vi "PDHydra - PWM_v2.vi"(8 "error in":errorcluster, 9 "Board Selector":T1, 10 "HMP VISA":refnum<visa-resource-name>="HMP4040_FTS2", 11 "ControlBoardVISA":refnum<visa-resource-name>="ControlBoard") -> (0 "error out":errorcluster, 1 "50% Duty Cycle":dbl[](array[numeric]), 2 "25% Duty":dbl[](array[numeric]), 3 "0% Duty":dbl[](array[numeric]))   [LabVIEW 2022 SP3]
uses:
  Serial Board Com/Board Select.ctl
  Serial Board Com/ADCSelector BB.ctl
  HMP4000 Communication/HMP4040_ChannelControlAutomatic.ctl
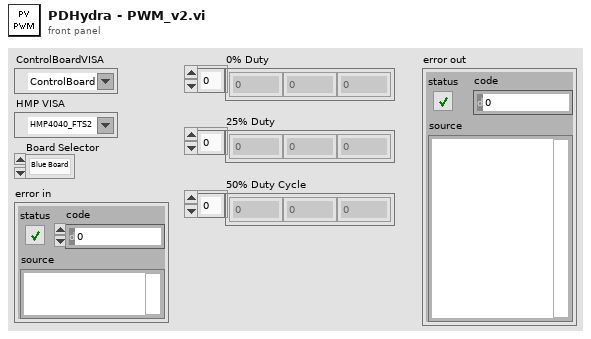
[diagram p1: front panel]
types:
  T1 = typedef "Board Select.ctl" = enum16{"Blue Board", "Green Board"}
  T2 = typedef "HMP4040_ChannelControlAutomatic.ctl" = enum16{"Off", "Control Power", "HMP2020 Control + DC32V", "HMP2020 Control + DC8V", "HMP4040 Control + DC32V", "HMP4040 Control +DC8V", "HMP4040 Ch2 24V 4A"}
  T3 = typedef "ADCSelector BB.ctl" = enum16{"INVA_ISENSE_U", "INVA_ISENSE_V", "INVA_ISENSE_W", "INVA_UDC", "INVA_TEMP", "HB_TEMP", "AUXB_TEMP", "VLINE_AB", "VLINE_BC", "VLINE_CA", "VSENSE_POS_24V", "VSENSE_POS_5V", "VSENSE_NEG_15V", "INVB_ISENSE_U", "INV_B_ISENSEV", "INVB_ISENSE_W", "INVB_UDC", "INVB_TEMP", "AUXA_TEMP", "AUXC_TEMP", "VOUT_AB", "VOUT_BC", "VOUT_CA", "VSENSE_POS_15V", "VSENSE_POS_3P3V", "TEST_POINT"}
  T4 = cluster{"Enum":T3, "Duty Cycle On":i32, "Leg":i32, "Duty Cycle Off":i32}[]
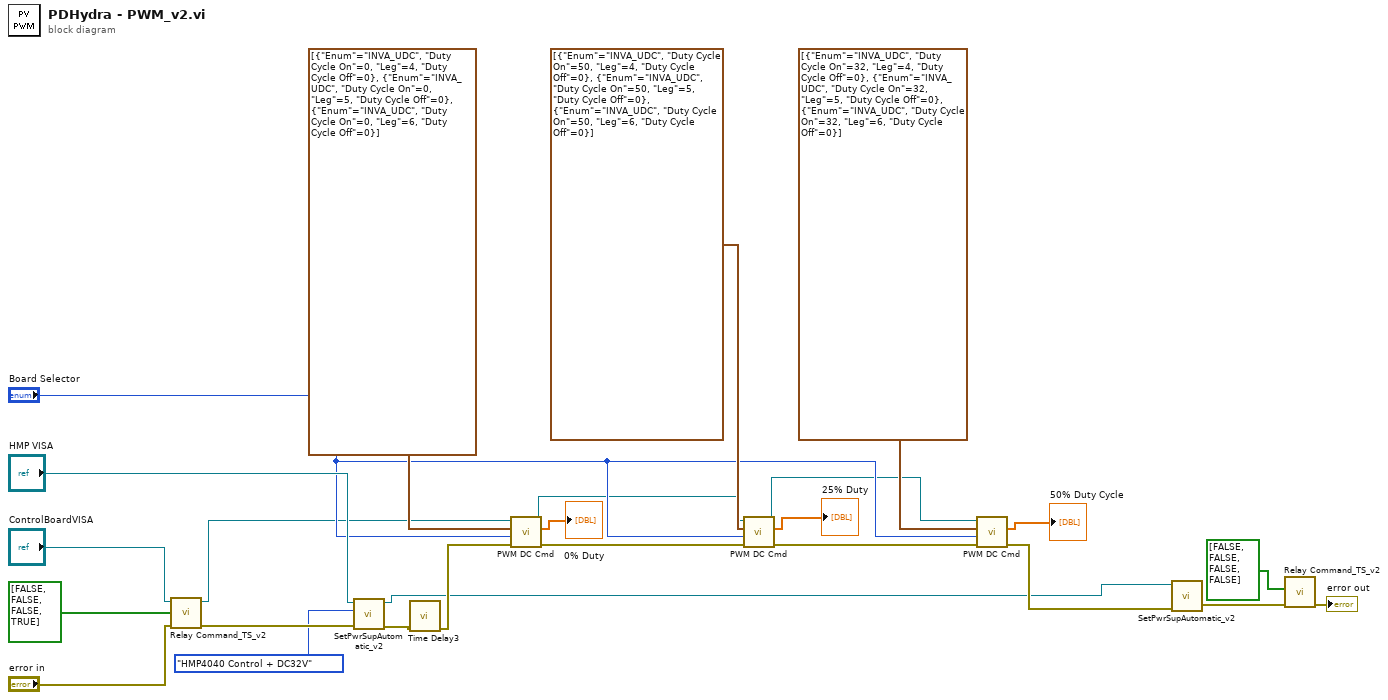
[diagram p0: block diagram]
diagram:
  n1 = call "Relay Command_TS_v2.vi"("error in (no error)"="error in", "Relay Command"=bool[] [FALSE, FALSE, FALSE, TRUE], "Control Board VISA"="ControlBoardVISA") -> ("error out"=w22:errorcluster, "VISA Refnum out"=w8:refnum<visa-resource-name>)  [unwired: 7 in]
  n2 = call "SetPwrSupAutomatic_v2.vi"("error in (no error)"=w22, "Enum"=HMP4040_ChannelControlAutomatic."HMP4040 Control + DC32V", "HMP VISA"="HMP VISA") -> ("error out"=w21:errorcluster, "HMP VISA Out"=w7:refnum<visa-resource-name>)  [unwired: 7 in]
  n3 = call "Time Delay3"("error in (no error)"=w21) -> ("error out"=w17:errorcluster)  [unwired: 10 in]
  n4 = call "PWM DC Cmd.vi"("error in (no error)"=w17, "Board Selector"="Board Selector", "Array in"=T4 [{"Enum"=enum."INVA_UDC", "Duty Cycle On"=0, "Leg"=4, "Duty Cycle Off"=0}, {"Enum"=enum."INVA_UDC", "Duty Cycle On"=0, "Leg"=5, "Duty Cycle Off"=0}, {"Enum"=enum."INVA_UDC", "Duty Cycle On"=0, "Leg"=6, "Duty Cycle Off"=0}], "VISA Refnum in"=w8) -> ("error out"=w19:errorcluster, "Array out"=→"0% Duty":dbl[], "VISA Refnum out"=w4:refnum<visa-resource-name>)  [unwired: 5 in]
  n5 = call "PWM DC Cmd.vi"("error in (no error)"=w19, "Board Selector"="Board Selector", "Array in"=T4 [{"Enum"=enum."INVA_UDC", "Duty Cycle On"=50, "Leg"=4, "Duty Cycle Off"=0}, {"Enum"=enum."INVA_UDC", "Duty Cycle On"=50, "Leg"=5, "Duty Cycle Off"=0}, {"Enum"=enum."INVA_UDC", "Duty Cycle On"=50, "Leg"=6, "Duty Cycle Off"=0}], "VISA Refnum in"=w4) -> ("error out"=w15:errorcluster, "Array out"=→"25% Duty":dbl[], "VISA Refnum out"=w3:refnum<visa-resource-name>)  [unwired: 5 in]
  n6 = call "PWM DC Cmd.vi"("error in (no error)"=w15, "Board Selector"="Board Selector", "Array in"=T4 [{"Enum"=enum."INVA_UDC", "Duty Cycle On"=32, "Leg"=4, "Duty Cycle Off"=0}, {"Enum"=enum."INVA_UDC", "Duty Cycle On"=32, "Leg"=5, "Duty Cycle Off"=0}, {"Enum"=enum."INVA_UDC", "Duty Cycle On"=32, "Leg"=6, "Duty Cycle Off"=0}], "VISA Refnum in"=w3) -> ("error out"=w11:errorcluster, "Array out"=→"50% Duty Cycle":dbl[])  [unwired: 5 in, 1 out]
  n7 = call "SetPwrSupAutomatic_v2.vi"("error in (no error)"=w11, "HMP VISA"=w7) -> ("error out"=w14:errorcluster)  [unwired: 8 in, 1 out]
  n8 = call "Relay Command_TS_v2.vi"("error in (no error)"=w14, "Relay Command"=bool[] [FALSE, FALSE, FALSE, FALSE]) -> ("error out"=→"error out":errorcluster)  [unwired: 8 in, 1 out]
